vi "mecanum_set_outputs.vi"(11 "Mecanum":T1) -> ()   [LabVIEW 2012]
uses:
  mecanum_output.ctl
  <vilib>/Rock Robotics/WPI/CAN/Jaguar/SubVIs/WPI_CANJaguar_StatusSelect.ctl
panel:
  out "X Position":dbl
  out "Y Position":dbl
  out "Position Front Left":dbl
  out "Position Front Right":dbl
  out "Position Back Right":dbl
  out "Position Back Left":dbl
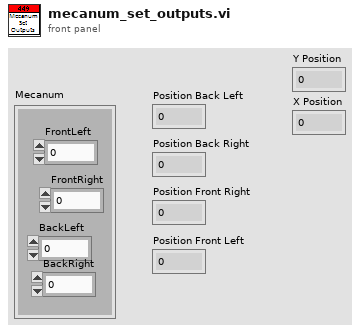
[diagram p1: front panel]
types:
  T1 = typedef "mecanum_output.ctl" = cluster{"FrontLeft":dbl, "FrontRight":dbl, "BackLeft":dbl, "BackRight":dbl}
  T2 = typedef "WPI_CANJaguar_StatusSelect.ctl" = enum16{"Output Percent VBus", "Output Voltage", "Bus Voltage", "Current", "Temperature", "Position", "Speed", "Limit Switches", "Faults", "Fault Counters", "Power Cycle"}
  T3 = typedef "WPI_MotorControlDeviceRef.ctl" = cluster{"DeviceStatus":errorcluster, "Type":enum16{"PWM", "CAN"}, "PWM":cluster{"Digital Module":T4, "PWM Channel":T5, "DeadBand":T6}, "CAN":cluster{"Device Number":u8, "Control Mode":T7, "Semaphore":T8, "Max Vout":dbl}, "Invert":bool, "TransformRef":T9, "InvTransformRef":T9}
  T4 = typedef "FPGA_TypedefDigitalModule.ctl" = enum16{"Digital Module 1", "Digital Module 2"}
  T5 = typedef "FPGA_DIOPWMChannel.ctl" = enum8{"PWM 1", "PWM 2", "PWM 3", "PWM 4", "PWM 5", "PWM 6", "PWM 7", "PWM 8", "PWM 9", "PWM 10", "Invalid"}
  T6 = typedef "WPI_PWMDeadband.ctl" = cluster{"Name":string, "maxPositivePwm":i32, "minPositivePwm":i32, "centerPwm":i32, "maxNegativePwm":i32, "minNegativePwm":i32, "angularRange":u16}
  T7 = typedef "WPI_CANJaguar_ControlMode.ctl" = enum8{"Percent VBus", "Current", "Speed", "Position", "Voltage"}
  T8 = typedef "Semaphore RefNum" = refnum<k1>
  T9 = typedef "WPI_PWMTransform_ConPane.ctl" = refnum<vi>
  T10 = typedef "WPI_CANJaguar_Status.ctl" = cluster{"Output Percent VBus":dbl, "Output Voltage":dbl, "Bus Voltage":dbl, "Current":dbl, "Temperature":dbl, "Position":dbl, "Speed":dbl, "Limits":cluster{"Forward Limit":bool, "Reverse Limit":bool, "Forward Soft Limit":bool, "Reverse Soft Limit":bool, "Sticky Forward Limit":bool, "Sticky Reverse Limit":bool, "Sticky Forward Soft Limit":bool, "Sticky Reverse Soft Limit":bool}, "Faults":cluster{"Current Fault":bool, "Temperature Fault":bool, "Bus Voltage Fault":bool, "Gate Driver Fault":bool, "Comm Fault":bool}, "Fault Counters":cluster{"Current Faults":u8, "Temperature Faults":u8, "Bus Voltage Faults":u8, "Gate Driver Faults":u8, "Comm Faults":u8, "CAN Status":u8, "CAN RX Errors":u8, "CAN TX Errors":u8}, "Power Cycle":bool}
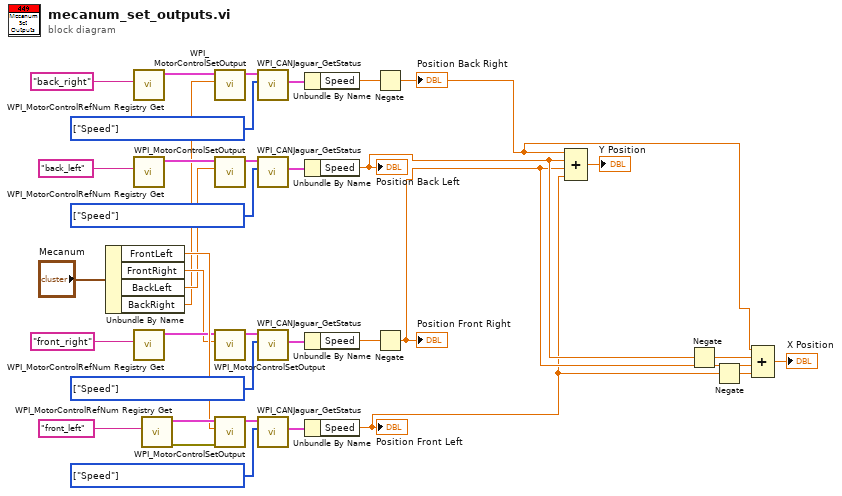
[diagram p0: block diagram]
diagram:
  w9 = T2[] [enum."Speed"] items=["Output Percent VBus", "Output Voltage", "Bus Voltage", "Current", "Temperature", "Position", "Speed", "Limit Switches", "Faults", "Fault Counters", "Power Cycle"] ("Status Select")
  w12 = T2[] [enum."Speed"] items=["Output Percent VBus", "Output Voltage", "Bus Voltage", "Current", "Temperature", "Position", "Speed", "Limit Switches", "Faults", "Fault Counters", "Power Cycle"] ("Status Select")
  w16 = T2[] [enum."Speed"] items=["Output Percent VBus", "Output Voltage", "Bus Voltage", "Current", "Temperature", "Position", "Speed", "Limit Switches", "Faults", "Fault Counters", "Power Cycle"] ("Status Select")
  w22 = T2[] [enum."Speed"] items=["Output Percent VBus", "Output Voltage", "Bus Voltage", "Current", "Temperature", "Position", "Speed", "Limit Switches", "Faults", "Fault Counters", "Power Cycle"] ("Status Select")
  n1 = Unbundle By Name("Mecanum") -> ("FrontLeft"=w33:dbl, "FrontRight"=w29:dbl, "BackLeft"=w26:dbl, "BackRight"=w23:dbl)
  n2 = call <vilib>:"WPI_MotorControlRefNum Registry Get.vi"("refnum name"="back_right") -> ("MotorControlDevRef"=w25:T3)  [unwired: 9 in, 1 out]
  n3 = call <vilib>:"WPI_MotorControlRefNum Registry Get.vi"("refnum name"="back_left") -> ("MotorControlDevRef"=w28:T3)  [unwired: 9 in, 1 out]
  n4 = call <vilib>:"WPI_MotorControlRefNum Registry Get.vi"("refnum name"="front_right") -> ("MotorControlDevRef"=w31:T3)  [unwired: 9 in, 1 out]
  n5 = call <vilib>:"WPI_MotorControlRefNum Registry Get.vi"("refnum name"="front_left") -> ("error out"=w32:errorcluster, "MotorControlDevRef"=w34:T3)  [unwired: 9 in]
  n6 = call <vilib>:"WPI_MotorControlSetOutput.vi"("Output"=w23, "MotorControlDevRef"=w25) -> ("MotorControlDevRef"=w17:T3)  [unwired: 7 in, 2 out]
  n7 = call <vilib>:"WPI_MotorControlSetOutput.vi"("Output"=w26, "MotorControlDevRef"=w28) -> ("MotorControlDevRef"=w20:T3)  [unwired: 7 in, 2 out]
  n8 = call <vilib>:"WPI_MotorControlSetOutput.vi"("Output"=w29, "MotorControlDevRef"=w31) -> ("MotorControlDevRef"=w13:T3)  [unwired: 7 in, 2 out]
  n9 = call <vilib>:"WPI_MotorControlSetOutput.vi"("error in (no error)"=w32, "Output"=w33, "MotorControlDevRef"=w34) -> ("MotorControlDevRef"=w10:T3)  [unwired: 6 in, 2 out]
  n10 = call <vilib>:"WPI_CANJaguar_GetStatus.vi"("Status Select"=w16, "CAN Jaguar Ref"=w17) -> ("Status"=w19:T10)  [unwired: 7 in, 2 out]
  n11 = call <vilib>:"WPI_CANJaguar_GetStatus.vi"("Status Select"=w22, "CAN Jaguar Ref"=w20) -> ("Status"=w21:T10)  [unwired: 7 in, 2 out]
  n12 = call <vilib>:"WPI_CANJaguar_GetStatus.vi"("Status Select"=w12, "CAN Jaguar Ref"=w13) -> ("Status"=w15:T10)  [unwired: 7 in, 2 out]
  n13 = call <vilib>:"WPI_CANJaguar_GetStatus.vi"("Status Select"=w9, "CAN Jaguar Ref"=w10) -> ("Status"=w11:T10)  [unwired: 7 in, 2 out]
  n14 = Unbundle By Name(w19) -> ("Speed"=w18:dbl)
  n15 = Unbundle By Name(w21) -> ("Speed"=w7:dbl)
  "Position Back Left" <- w7
  n16 = Unbundle By Name(w15) -> ("Speed"=w14:dbl)
  n17 = Unbundle By Name(w11) -> ("Speed"=w5:dbl)
  "Position Front Left" <- w5
  n18 = Negate(x=w18) -> (-x=w2:dbl)
  "Position Back Right" <- w2
  n19 = Negate(x=w14) -> (-x=w6:dbl)
  "Position Front Right" <- w6
  n20 = Compound Arithmetic op=ADD(w2, w7, w6, w5) -> (→"Y Position":dbl)
  n21 = Negate(x=w7) -> (-x=w1:dbl)
  n22 = Negate(x=w5) -> (-x=w4:dbl)
  n23 = Compound Arithmetic op=ADD(w2, w1, w6, w4) -> (→"X Position":dbl)
